vi "Cancel Async.vi"(7 "error in (no error)":errorcluster, 10 "DeviceRefnum":u64) -> (0 "error out":errorcluster, 3 "DeviceRefnum Out":u64)   [LabVIEW 2014]
panel:
  out "function return":i32
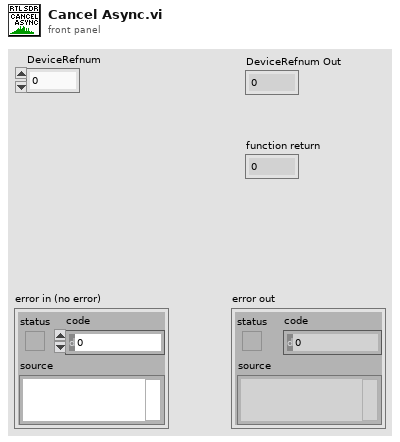
[diagram p1: front panel]
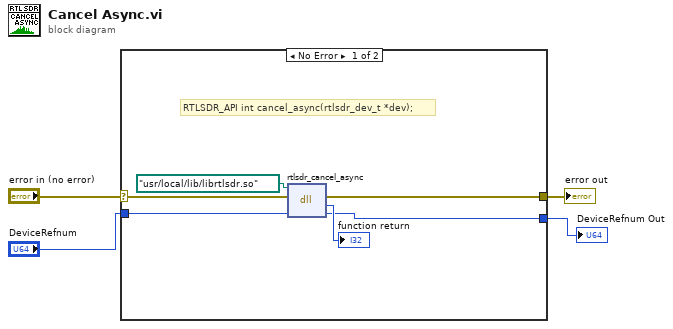
[diagram p0: block diagram]
diagram:
  n1 = case shown="No Error" "error in (no error)" {
    selector: "error in (no error)" -> [w8 w12]
    tunnel: [w7 w12] -> w4
    tunnel: "DeviceRefnum" -> [w10 w11]
    tunnel: [w5 w11] -> w1
    frame No Error {
      # "RTLSDR_API int cancel_async(rtlsdr_dev_t *dev);"
      n2 = dll-call lib="C:/Program Files (x86)/National Instruments/LabVIEW 2016/vi.lib/rtlsdr/rtlsdr.*" fn="rtlsdr_cancel_async"(path in=path "/usr/local/lib/librtlsdr.so", error in=w8, "DeviceRefnum"=w10) -> (error out=w7:errorcluster, "return type"=→"function return":i32, "DeviceRefnum"=w5:u64)  [unwired: 1 in, 1 out]
    }
    frame Error {
    }
  }
  "error out" <- w4
  "DeviceRefnum Out" <- w1
